vi "Build High Priority Check.vi"(6 "Group":i32, 7 "Virtual Memory Unit in":refnum<class "Virtual Memory Unit.lvclass">, 8 "error in (no error)":errorcluster, 10 "Starting Address":u16 format="%04x", 11 "Major Frame in":refnum<class "Major Frame.lvclass">) -> (0 "error out":errorcluster, 2 "Next Available Address":u16 format="%04x", 3 "Major Frame out":refnum<class "Major Frame.lvclass">, 5 "Virtual Memory Unit out":refnum<class "Virtual Memory Unit.lvclass">)   [LabVIEW 2020, in "BCI-1553 API.lvlib" / "Major Frame.lvclass"]
doc: "Builds a asynchronous high priority check instruction set.\n\nThis command set is triggerable by GP2, GP3, or GP4, depending on the group.\n\nGroup 0: GP2\nGroup 1: GP3\nGroup 2: GP4"
uses:
  Major Frame.lvclass
  Dependencies/Virtual Memory Unit/Virtual Memory Unit.lvclass
  TypeDefs/BC Op Codes - Verbose.ctl
  TypeDefs/BC Condition Codes.ctl
  Major Frame.lvclass/Major Frame.ctl
  BCI-1553 API.lvlib
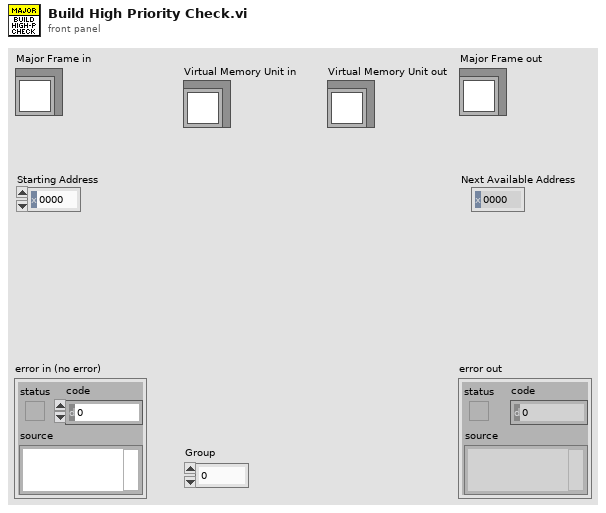
[diagram p1: front panel]
types:
  T1 = typedef "BCI-1553 API.lvlib/BC Condition Codes.ctl" = enum16{"GP0 == 1 || LT", "GP1 == 1 || NE", "GP2 == 1", "GP3 == 1", "GP4 == 1", "GP5 == 1", "GP6 == 1", "GP7 == 1", "NORESP", "FMTERR", "GOODBLOCK", "MSKSTATSET", "BADMSG", "1RETRY", "2RETRY", "ALWAYS"}
  T2 = typedef "BCI-1553 API.lvlib/BC Op Codes - Verbose.ctl" = enum16{"EXECUTE MSG", "EXECUTE MSG GO", "JUMP", "CALL SUBROUTINE", "RETURN", "INTERRUPT REQUEST", "HALT", "DELAY", "WAIT FRAME TIMER = 0", "COMPARE FRAME TIMER", "COMPARE MSG TIMER", "LOAD TIME TAG CTR", "LOAD TIME TAG CTR HI", "LOAD FRAME TIMER", "START FRAME TIMER", "PUSH TIME TAG COUNT", "PUSH TIME TAG COUNT HI", "PUSH TIME TAG COUNT BOTH", "PUSH BLOCK STATUS WORD", "PUSH CURRENT VALUE", "PUSH INDIRECT", "WAIT EXT TRIGGER", "EXECUTE AND FLIP", "EXECUTE, FLIP, GO", "WRITE VALUE TO WMI", "WRITE VALUE TO MEM", "DECREMENT RAM, SKIP", "FLAG"}
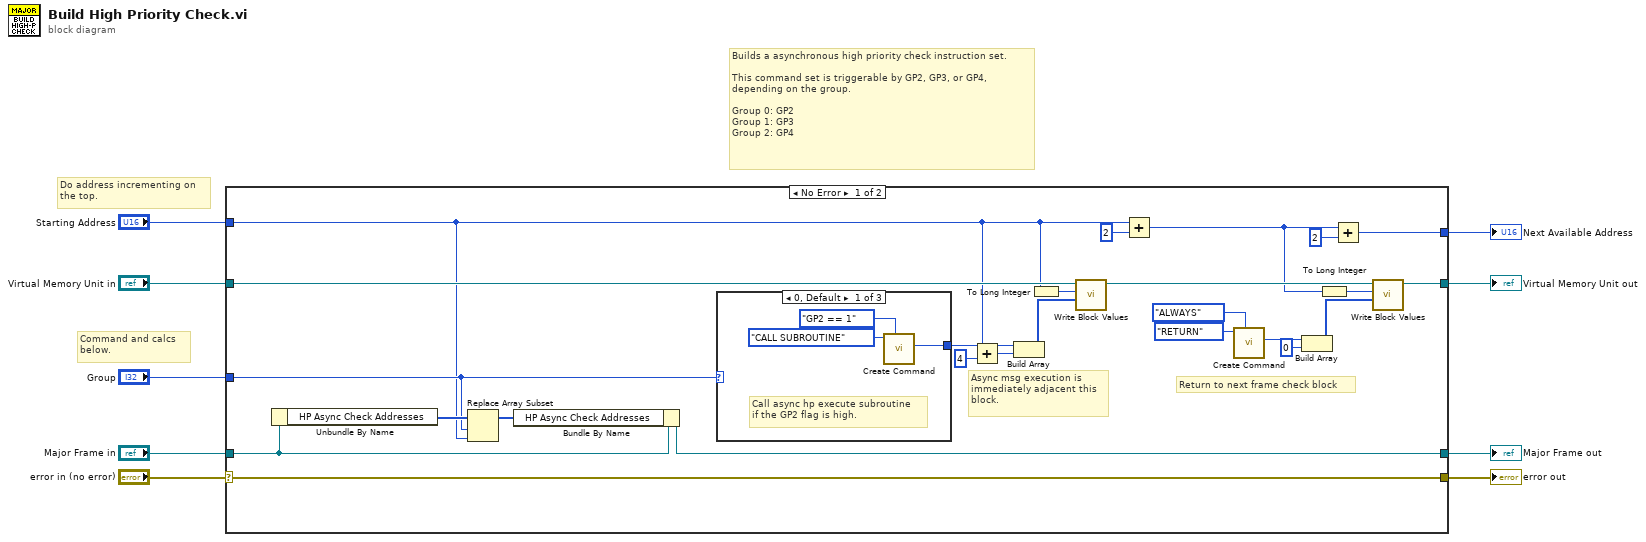
[diagram p0: block diagram]
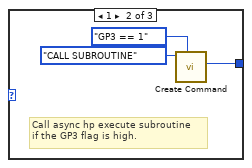
[diagram p2: hidden frame]
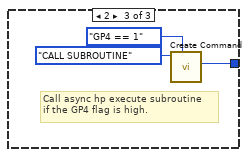
[diagram p3: hidden frame]
diagram:
  # "Command and calcs\nbelow."
  # "Do address incrementing on\nthe top."
  # "Builds a asynchronous high priority check instruction set.\n\nThis command set is triggerable by GP2, GP3, or GP4,\ndepending on the group.\n\nGroup 0: GP2\nGroup 1: GP3\nGroup 2: GP4"
  n1 = case shown="No Error" "error in (no error)" {
    selector: "error in (no error)" -> [w34 w45]
    tunnel: [w34 w45] -> w8
    tunnel: [w17 w44] -> w6
    tunnel: "Major Frame in" -> [w18 w44]
    tunnel: "Virtual Memory Unit in" -> [w33 _]
    tunnel: [w23 _] -> w4
    tunnel: "Starting Address" -> [w13 _]
    tunnel: "Group" -> [w14 _]
    tunnel: [w12 _] -> w1
    frame No Error {
      # "Async msg execution is\nimmediately adjacent this\nblock."
      # "Return to next frame check block"
      n2 = Unbundle By Name(w18) -> ("HP Async Check Addresses"=w16:u16[])
      n3 = Replace Array Subset(array=w16, new element=w13, index=w14) -> (w15:u16[])
      n4 = Bundle By Name(cluster=w18, "HP Async Check Addresses"=w15) -> (w17:refnum<class "Major Frame.lvclass">)
      n5 = case shown="0, Default" w14 {
        tunnel: [w35 w38 w41] -> w32
        frame 0, Default {
          # "Call async hp execute subroutine\nif the GP2 flag is high."
          n6 = call "Create Command.vi"("Condition"=BC_Condition_Codes."GP2 == 1", "Op Code"=BC_Op_Codes_-_Verbose."CALL SUBROUTINE") -> ("Instruction"=w35:u16)  [unwired: 8 in, 1 out]
        }
        frame 1 {
          # "Call async hp execute subroutine\nif the GP3 flag is high."
          n7 = call "Create Command.vi"("Condition"=BC_Condition_Codes."GP3 == 1", "Op Code"=BC_Op_Codes_-_Verbose."CALL SUBROUTINE") -> ("Instruction"=w38:u16)  [unwired: 8 in, 1 out]
        }
        frame 2 {
          # "Call async hp execute subroutine\nif the GP4 flag is high."
          n8 = call "Create Command.vi"("Condition"=BC_Condition_Codes."GP4 == 1", "Op Code"=BC_Op_Codes_-_Verbose."CALL SUBROUTINE") -> ("Instruction"=w41:u16)  [unwired: 8 in, 1 out]
        }
      }
      n9 = Add(x=w13, y=u16 4 ("x")) -> (x+y=w11:u16)
      n10 = Build Array(w32, w11) -> (w31:u16[])
      n11 = To Long Integer(number=w13) -> (32bit integer=w30:i32)
      n12 = call "Write Block Values.vi"("Write Block"=w31, "Start Index"=w30, "Virtual Memory Unit in"=w33) -> ("Virtual Memory Unit out"=w24:refnum<class "Virtual Memory Unit.lvclass">)  [unwired: 7 in, 1 out]
      n13 = Add(x=w13, y=u16 2) -> (x+y=w19:u16)
      n14 = call "Create Command.vi"("Condition"=BC_Condition_Codes."ALWAYS", "Op Code"=BC_Op_Codes_-_Verbose."RETURN") -> ("Instruction"=w22:u16)  [unwired: 8 in, 1 out]
      n15 = Build Array(w22, u16 0 ("element")) -> (w26:u16[])
      n16 = To Long Integer(number=w19) -> (32bit integer=w25:i32)
      n17 = Add(x=w19, y=u16 2) -> (x+y=w12:u16)
      n18 = call "Write Block Values.vi"("Write Block"=w26, "Start Index"=w25, "Virtual Memory Unit in"=w24) -> ("Virtual Memory Unit out"=w23:refnum<class "Virtual Memory Unit.lvclass">)  [unwired: 7 in, 1 out]
    }
    frame Error {
    }
  }
  "error out" <- w8
  "Major Frame out" <- w6
  "Next Available Address" <- w1
  "Virtual Memory Unit out" <- w4
